vi "Get MAC&SN.vi"(8 "error in (no error)":errorcluster caption="错误输入（无错误）", 11 "MAC&SN":string) -> (0 "error out":errorcluster caption="错误输出", 2 "mac":string, 3 "sn":string)   [LabVIEW 2012]
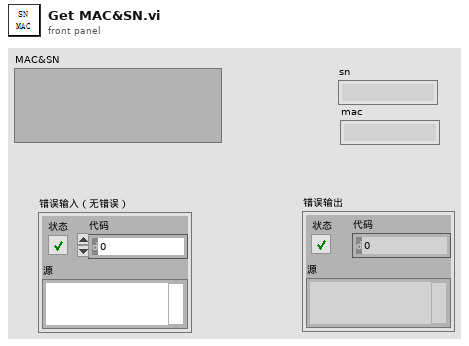
[diagram p1: front panel]
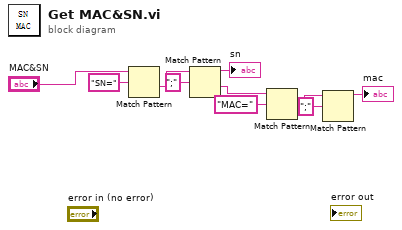
[diagram p0: block diagram]
diagram:
  n1 = Match Pattern(string="MAC&SN", regular expression="SN=" ("正则表达式")) -> (after substring=w8:string)  [unwired: 1 in, 3 out]
  n2 = Match Pattern(string=w8, regular expression=";" ("正则表达式")) -> (before substring=→"sn":string, after substring=w5:string)  [unwired: 1 in, 2 out]
  n3 = Match Pattern(string=w5, regular expression="MAC=" ("正则表达式")) -> (after substring=w3:string)  [unwired: 1 in, 3 out]
  n4 = Match Pattern(string=w3, regular expression=";" ("正则表达式")) -> (before substring=→"mac":string)  [unwired: 1 in, 3 out]
